vi "pa to list.vi"(8 "x end":dbl, 9 "x start":dbl, 10 "b":dbl, 11 "K":dbl) -> (2 "F-format string":string[][](array[string]), 3 "array":dbl[][](array[numeric]))   [LabVIEW 2011]
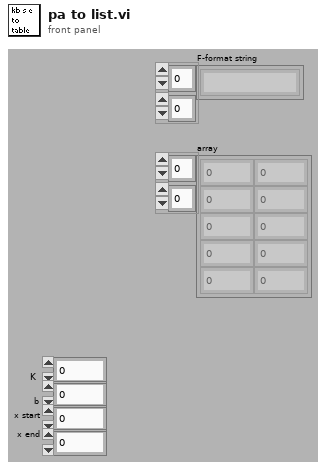
[diagram p1: front panel]
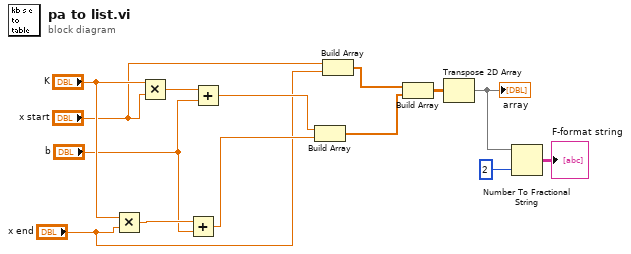
[diagram p0: block diagram]
diagram:
  n1 = Multiply(x="K", y="x end") -> (x*y=w12:dbl)
  n2 = Multiply(x="K", y="x start") -> (x*y=w14:dbl)
  n3 = Add(x=w12, y="b") -> (x+y=w9:dbl)
  n4 = Add(x=w14, y="b") -> (x+y=w10:dbl)
  n5 = Build Array(w10, w9) -> (w5:dbl[])
  n6 = Build Array("x start", "x end") -> (w6:dbl[])
  n7 = Build Array(w6, w5) -> (w4:dbl[][])
  n8 = Transpose 2D Array(2D array=w4) -> (transposed array=w2:dbl[][])
  "array" <- w2
  n9 = Number To Fractional String(number=w2, precision (6)=i16 2) -> (F-format string=→"F-format string":string[][])  [unwired: 2 out]
